vi "strings.vi"() -> ()   [LabVIEW 2012]
panel:
  out "replaced substring":string
  out "result string":string
  out "substring":string
  out "length":i32
  in  "String 2":string
  in  "String":string
  out "concatenated string":string
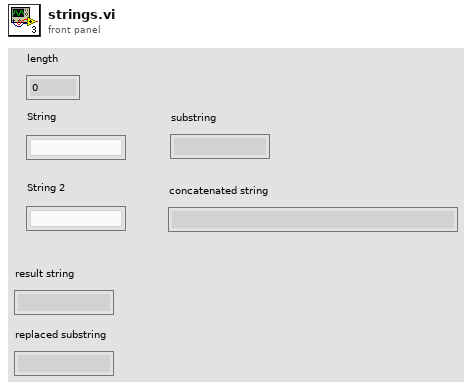
[diagram p1: front panel]
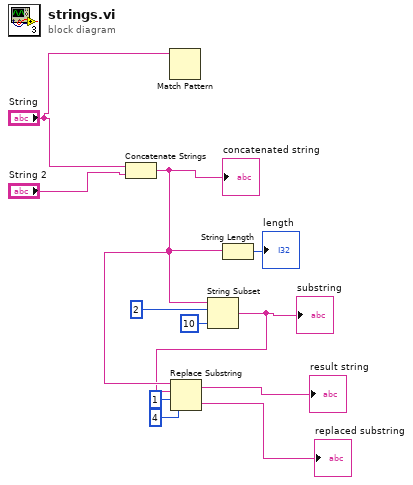
[diagram p0: block diagram]
diagram:
  n1 = Concatenate Strings("String", "String 2") -> (w5:string)
  "concatenated string" <- w5
  n2 = Match Pattern(string="String") -> ()  [unwired: 2 in, 4 out]
  n3 = String Subset(string=w5, offset (0)=2, length (rest)=10 ("length (rest)")) -> (substring=w4:string)
  "substring" <- w4
  n4 = Replace Substring(2:4 ("length (len. of substring)"), 3:1 ("offset (0)"), 4:w4, 5:w5) -> (0:→"replaced substring":string, 1:→"result string":string)
  n5 = String Length(string=w5) -> (length=→"length":i32)
